vi "insert.vi"(8 "error in (no error)":errorcluster, 11 "IntrinsicImagingMG091001 in":refnum<class "DataCollectionMG091001IntrinsicImaging.lvclass">) -> (0 "error out":errorcluster, 3 "IntrinsicImagingMG091001 out":refnum<class "DataCollectionMG091001IntrinsicImaging.lvclass">)   [LabVIEW 2010, in "DataCollectionMG091001IntrinsicImaging.lvclass"]
uses:
  DataCollectionMG091001IntrinsicImaging.lvclass
  common/classes/Image/Image/Image.lvclass
  DataCollectionMG091001IntrinsicImaging.lvclass/DataCollectionMG091001IntrinsicImaging.ctl
  common/classes/ErrorController/ErrorController/class_data.vi
  common/classes/ErrorController/ErrorController/ErrorController.lvclass
  common/classes/ImageCollection/ImageCollection/ImageCollection.lvclass
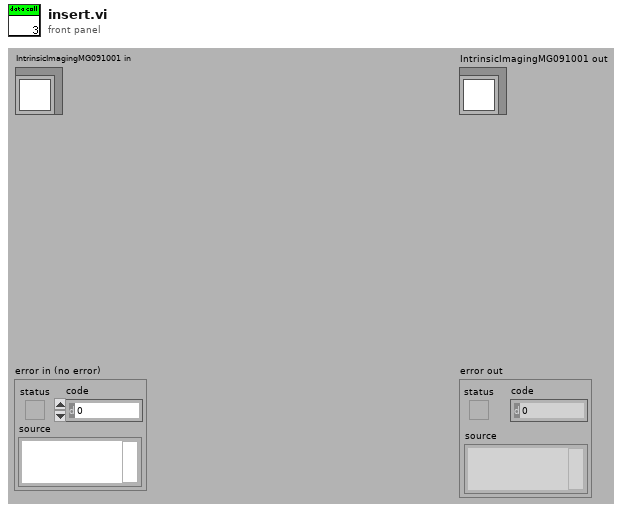
[diagram p1: front panel]
types:
  T1 = typedef "Image Type" = u32
  T2 = typedef "GenericToplevelComponent.lvclass/common_trigger_enum.ctl" = enum16{"NULL", "initialise", "terminate", "fetch command", "fetch data", "attach observer", "register as observer", "detach observer", "acknowledge", "start", "stop", "sweep started", "sweep finished", "experiment started", "experiment stopped"}
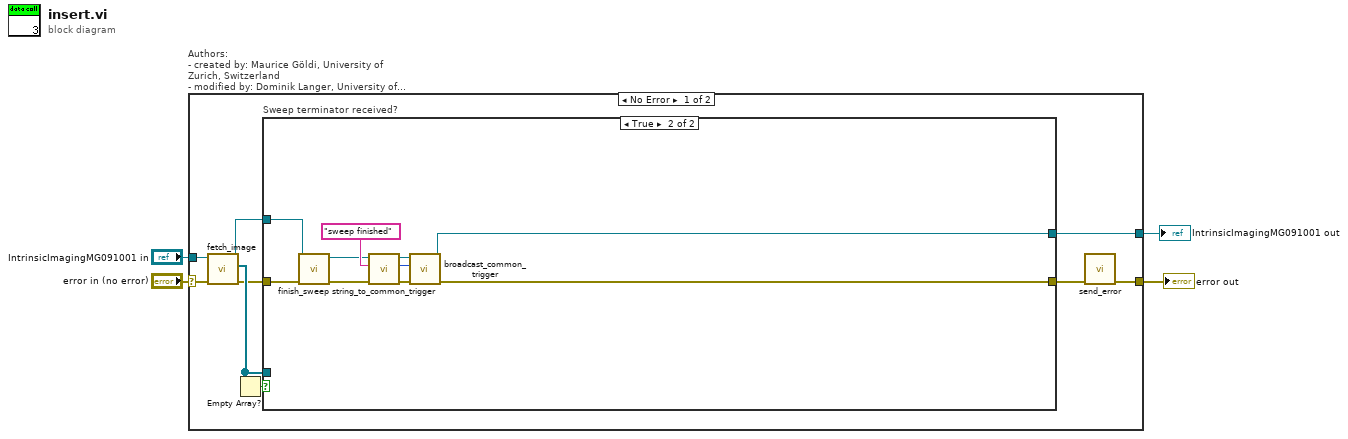
[diagram p0: block diagram]
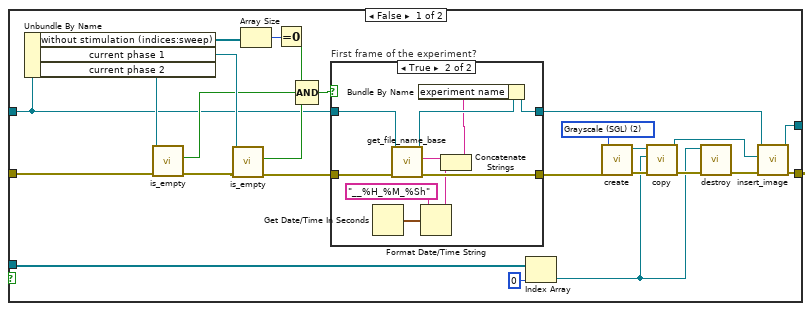
[diagram p2: hidden frame]
diagram:
  n1 = case "Authors: \n- created by: Maurice Göldi, University of Zurich, Switzerland\n- modified by: Dominik Langer, University of Zurich, Switzerland" shown="No Error" "error in (no error)" {
    selector: "error in (no error)" -> [w13 w62]
    tunnel: [w7 w62] -> w4
    tunnel: [w10 w61] -> w3
    tunnel: "IntrinsicImagingMG091001 in" -> [w12 w61]
    frame No Error {
      n2 = call-dynamic "fetch_image.vi"("error in (no error)"=w13, "GenericToplevelComponent in"=w12) -> ("error out"=w5:errorcluster, "image (channels)"=w8:refnum<class "Image.lvclass">[], "GenericToplevelComponent out"=w11:refnum<class "DataCollectionMG091001IntrinsicImaging.lvclass">)  [unwired: 4 in, 3 out]
      n3 = Empty Array?(array=w8) -> (empty?=w9:bool)
      n4 = case "Sweep terminator received?" shown="True" w9 {
        tunnel: [w38 w53] -> w6
        tunnel: w11 -> [w21 w59]
        tunnel: [w37 w51] -> w10
        tunnel: w8 -> [w36 _]
        tunnel: w5 -> [w26 w60]
        frame False {
          w31 = T1 2 items=["Grayscale (U8)", "Grayscale (I16)", "Grayscale (SGL)", "Complex (CSG)", "RGB (U32)", "HSL (U32)", "RGB (U64)", "Grayscale (U16)"] ("Image Type")
          n5 = Unbundle By Name(w21) -> ("without stimulation (indices:sweep)"=w16:refnum<class "ImageCollection.lvclass">[], "current phase 1"=w25:refnum<class "ImageCollection.lvclass">, "current phase 2"=w27:refnum<class "ImageCollection.lvclass">)
          n6 = call "is_empty.vi"("error in (no error)"=w26, "ImageCollection in"=w27) -> ("error out"=w24:errorcluster, "is empty?"=w23:bool)  [unwired: 7 in, 1 out]
          n7 = call "is_empty.vi"("error in (no error)"=w24, "ImageCollection in"=w25) -> ("error out"=w20:errorcluster, "is empty?"=w22:bool)  [unwired: 7 in, 1 out]
          n8 = Array Size(array=w16) -> (size(s)=w15:i32)
          n9 = Equal To 0?(x=w15) -> (x = 0?=w14:bool)
          n10 = Compound Arithmetic op=AND(w14, w23, w22) -> (w17:bool)
          n11 = case "First frame of the experiment?" shown="True" w17 {
            tunnel: w21 -> [w39 w50]
            tunnel: w20 -> [w40 w49]
            tunnel: [w40 w48] -> w19
            tunnel: [w39 w42] -> w18
            frame False {
            }
            frame True {
              n12 = Get Date/Time In Seconds() -> (seconds since 1Jan1904=w45:timestamp)
              n13 = call-dynamic "get_file_name_base.vi"("error in (no error)"=w49, "GenericComponent in"=w50) -> ("error out"=w48:errorcluster, "file name base"=w47:string, "GenericComponent out"=w43:refnum<class "DataCollectionMG091001IntrinsicImaging.lvclass">)  [unwired: 7 in]
              n14 = Format Date/Time String(time format string (%c)="__%H_%M_%Sh", seconds (now)=w45) -> (date/time string=w44:string)  [unwired: 1 in]
              n15 = Concatenate Strings(w47, w44) -> (w41:string)
              n16 = Bundle By Name(cluster=w43, "experiment name"=w41) -> (w42:refnum<class "DataCollectionMG091001IntrinsicImaging.lvclass">)
            }
          }
          n17 = Index Array(array=w36, index=0) -> (element=w28:refnum<class "Image.lvclass">)
          n18 = call "create.vi"("error in (no error)"=w19, "Image Type"=w31) -> ("error out"=w34:errorcluster, "Image out"=w29:refnum<class "Image.lvclass">)  [unwired: 8 in]
          n19 = call "copy.vi"("error in (no error)"=w34, "image to copy (source)"=w28, "Image in (target)"=w29) -> ("error out"=w33:errorcluster, "Image out"=w30:refnum<class "Image.lvclass">)  [unwired: 7 in]
          n20 = call-dynamic "destroy.vi"("error in (no error)"=w33, "Image in"=w28) -> ("error out"=w32:errorcluster)  [unwired: 8 in, 1 out]
          n21 = call-dynamic "insert_image.vi"("error in (no error)"=w32, "image"=w30, "DataCollectionMG091001IntrinsicImaging in"=w18) -> ("error out"=w38:errorcluster, "DataCollectionMG091001IntrinsicImaging out"=w37:refnum<class "DataCollectionMG091001IntrinsicImaging.lvclass">)  [unwired: 7 in]
        }
        frame True {
          n22 = call-dynamic "finish_sweep.vi"("error in (no error)"=w60, "DataCollectionMG091001IntrinsicImaging in"=w59) -> ("error out"=w54:errorcluster, "DataCollectionMG091001IntrinsicImaging out"=w52:refnum<class "DataCollectionMG091001IntrinsicImaging.lvclass">)  [unwired: 8 in]
          n23 = call-dynamic "string_to_common_trigger.vi"("error in (no error)"=w54, "trigger string"="sweep finished", "GenericToplevelComponent in"=w52) -> ("error out"=w57:errorcluster, "trigger"=w55:T2, "GenericToplevelComponent out"=w56:refnum<class "DataCollectionMG091001IntrinsicImaging.lvclass">)  [unwired: 6 in]
          n24 = call-dynamic "broadcast_common_trigger.vi"("error in (no error)"=w57, "trigger"=w55, "GenericToplevelComponent in"=w56) -> ("error out"=w53:errorcluster, "GenericToplevelComponent out"=w51:refnum<class "DataCollectionMG091001IntrinsicImaging.lvclass">)  [unwired: 7 in]
        }
      }
      n25 = call "send_error.vi"("error in (no error)"=w6) -> ("error out"=w7:errorcluster)  [unwired: 10 in]
    }
    frame Error {
    }
  }
  "error out" <- w4
  "IntrinsicImagingMG091001 out" <- w3
